vi "delay_sleep_deprivation_start.vi"(2 "Input \nparameters":T2={"Frame rate (ms)"=2000, "Worm strain"="N2", "Time t"=0, "State"=enum."Image acquisition", "Time elapsed"=0.0, "Max_num_runs"=100000, "#TTL"=0, "Time of start TTL"=100000, "ImSub Value"=0, "Time of last TTL"=0, "Number of Columns"=2, "Number of Rows"=2, "# AdjacentTTL"=0, "Sleep deprivation status"="", "Sleep Detection"=FALSE, "# Sleep detections"=0, "Time of first sleep detection"=0, "Time max # adjacent TTL"=0, "Image t-1"=[], "Image t"=[]} {"Number of Rows" items=["1"=1, "2"=2, "3"=3, "4"=4]; "Number of Columns" items=["1"=1, "2"=2, "3"=3, "4"=4]}, 3 "Deprivation\nparameters":T3={"Frame Row"=0, "Kstd"=40.0, "# Images for\nsleep detection"=10, "Kmean"=1.5, "Start time of sleep detection"=1000, 0, "Max deprivation length"=3600, "Max # TTL"=10000, "Delay detection start by x images after first detection"=0, "Minimum Interval between TTL pulses"=0, "Delay sleep detection\nby x detections"=9, "# Total immobility\n detections"=0.0, "Pause max # adjacent\nTTL"=0, "TTL x start\ntime deprivation\n"=0.0, "Max #\nadjacent TTL"=10000, " Ca2+\nmode"=0} {"?" items=["1", "2", "3", "4"]; "Frame Row" items=["1", "2", "3", "4"]}) -> (0 "Output \nparameters":T2={"Frame rate (ms)"=2000, "Worm strain"="N2", "Time t"=0, "State"=enum."Image acquisition", "Time elapsed"=0.0, "Max_num_runs"=100000, "#TTL"=0, "Time of start TTL"=100000, "ImSub Value"=0, "Time of last TTL"=0, "Number of Columns"=2, "Number of Rows"=2, "# AdjacentTTL"=0, "Sleep deprivation status"="", "Sleep Detection"=FALSE, "# Sleep detections"=0, "Time of first sleep detection"=0, "Time max # adjacent TTL"=0, "Image t-1"=[], "Image t"=[]} {"Number of Rows" items=["1"=1, "2"=2, "3"=3, "4"=4]; "Number of Columns" items=["1"=1, "2"=2, "3"=3, "4"=4]})   [LabVIEW 2011]
uses:
  state.ctl
panel:
  # "Sleep deprivation settings"
  # "Select deprivation animal"
  # "Deprive image in row"
  # "Deprive image in column"
  # "Sleep detection parameters"
  # "Sleep deprivation parameters"
  # "Delay deprivation start:"
  # "Pause deprivation (images):"
  # "Stop deprivation after:"
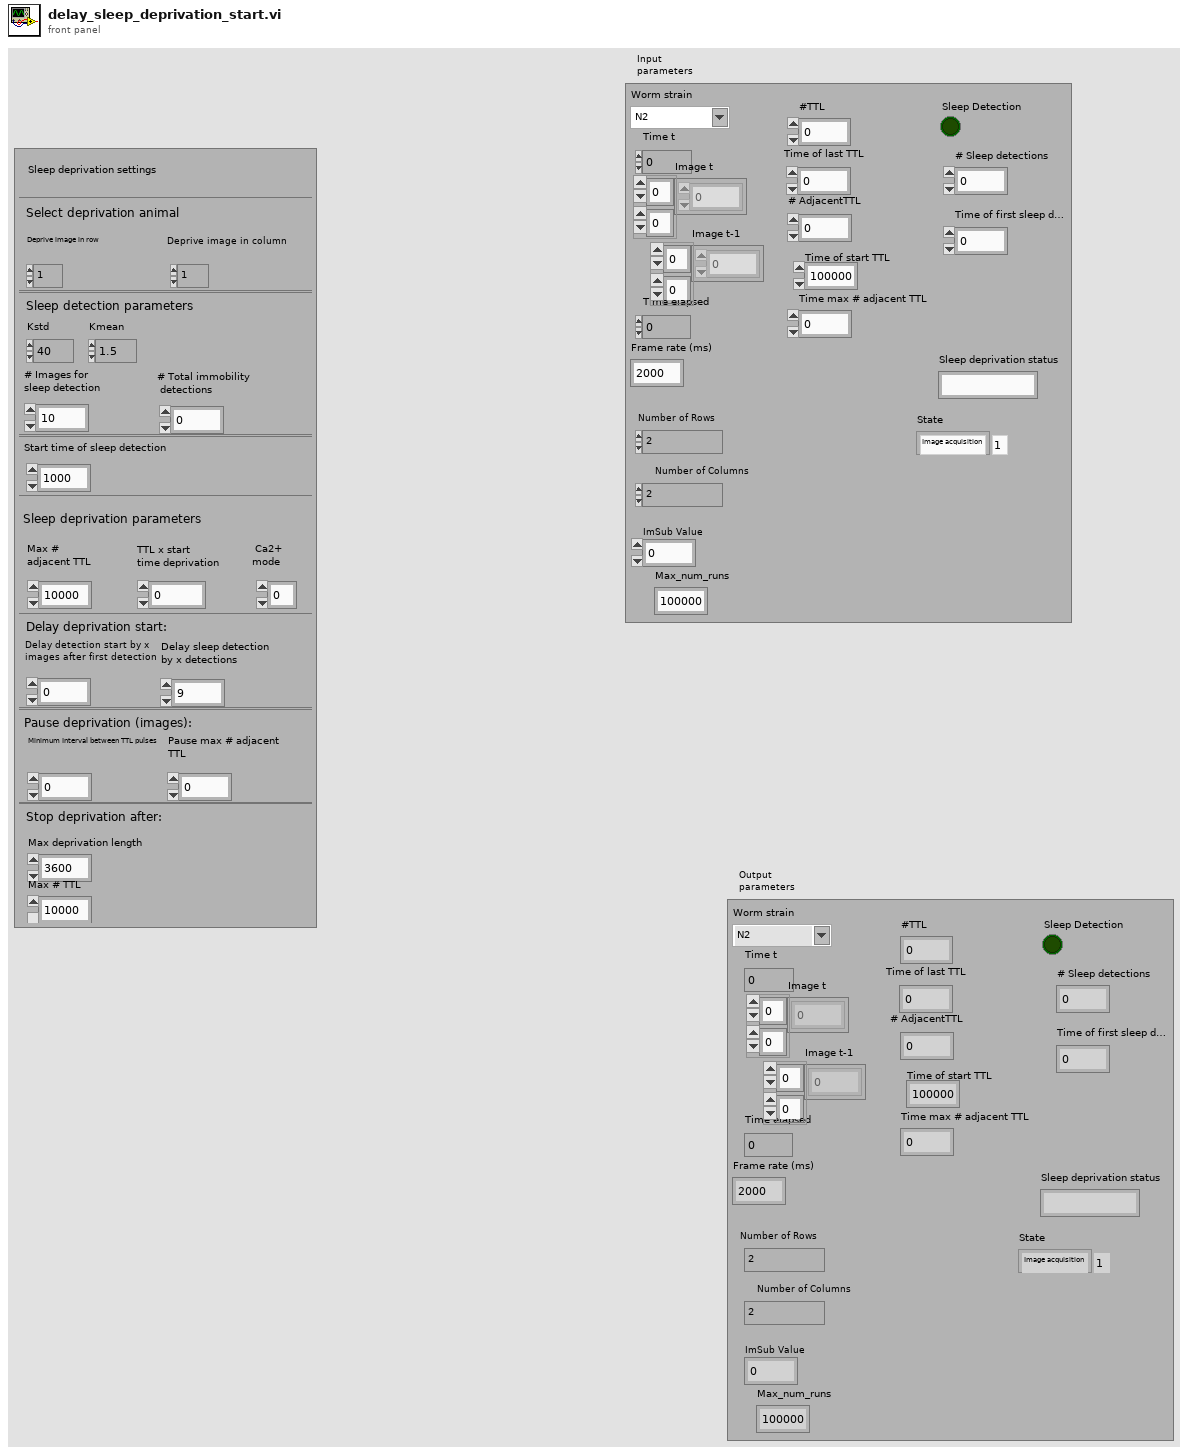
[diagram p1: front panel]
types:
  T1 = typedef "state.ctl" = enum16{"Initialize measurement", "Image acquisition", "Image processing", "Sleep detection", "Control TTL protocol ", "Sleep deprivation", "Update image & exit condition", "Wait "}
  T2 = cluster{"Frame rate (ms)":u32, "Worm strain":string, "Time t":i32, "State":T1, "Time elapsed":dbl, "Max_num_runs":i32, "#TTL":i32, "Time of start TTL":i32, "ImSub Value":i32, "Time of last TTL":i32, "Number of Columns":u32, "Number of Rows":u32, "# AdjacentTTL":i32, "Sleep deprivation status":string, "Sleep Detection":bool, "# Sleep detections":i32, "Time of first sleep detection":i32, "Time max # adjacent TTL":i32, "Image t-1":i32[][], "Image t":i32[][]}
  T3 = cluster{"Frame Row":u32, "Kstd":dbl, "# Images for\nsleep detection":i32, "Kmean":dbl, "Start time of sleep detection":i32, u32, "Max deprivation length":i32, "Max # TTL":i32, "Delay detection start by x images after first detection":i32, "Minimum Interval between TTL pulses":i32, "Delay sleep detection\nby x detections":i32, "# Total immobility\n detections":dbl, "Pause max # adjacent\nTTL":i32, "TTL x start\ntime deprivation\n":dbl, "Max #\nadjacent TTL":i32, " Ca2+\nmode":i32}
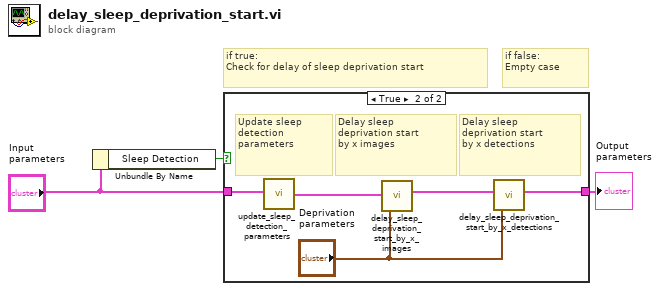
[diagram p0: block diagram]
diagram:
  # "if false: \nEmpty case"
  # "if true:\nCheck for delay of sleep deprivation start"
  n1 = Unbundle By Name("Input \nparameters") -> ("Sleep Detection"=w3:bool)
  n2 = case shown="True" w3 {
    tunnel: "Input \nparameters" -> [w4 w8]
    tunnel: [w4 w6] -> w2
    frame False {
    }
    frame True {
      # "Delay sleep\ndeprivation start\nby x detections"
      # "Delay sleep \ndeprivation start\nby x images"
      # "Update sleep\ndetection \nparameters"
      n3 = call "update_sleep_detection_parameters.vi"("Input \nparameters"=w8) -> ("Output \nParameters"=w7:T2)  [unwired: 4 in]
      n4 = call "delay_sleep_deprivation_start_by_x_images.vi"("Input \nParameters"=w7, "Deprivation\nparameters"="Deprivation\nparameters") -> ("Output \nParameters"=w9:T2)  [unwired: 6 in]
      n5 = call "delay_sleep_deprivation_start_by_x_detections.vi"("Deprivation\nparameters"="Deprivation\nparameters", "Input \nparameters"=w9) -> ("Output \nparameters"=w6:T2)  [unwired: 4 in]
    }
  }
  "Output \nparameters" <- w2
